vi "Run Action_Do.vi"(8 "error in (no error)":errorcluster, 10 "Project Builder in":refnum<class "Project Builder.lvclass">, 11 "Build Named Build Specification":refnum<class "Build Named Build Specification.lvclass">) -> (0 "error out":errorcluster, 1 "Success?":bool, 3 "Report":refnum<class "Report Data.lvclass">)   [LabVIEW 2019, in "ProjectBuilder.lvlib" / "Build Named Build Specification.lvclass"]
doc: "Run the action associated with the 'Project Action'-class.\n\nThis implementation builds a named build specification on the given target in the project."
uses:
  Build Named Build Specification.lvclass
  <vilib>/AppBuilder/AB_API_Simple/NI_App_Builder_API.lvlib
  Project Action/Project Action.lvclass
  Build Named Build Specification Data/Build Named Build Specification Data.lvclass
  <vilib>/AppBuilder/AB_API_Simple/Build (path).vi
  Data/Report Data/Report Data.lvclass
  Project Builder/Project Builder.lvclass
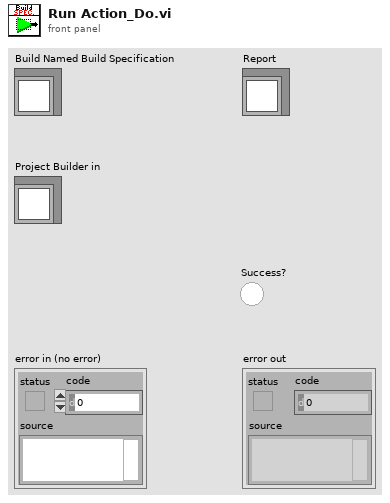
[diagram p1: front panel]
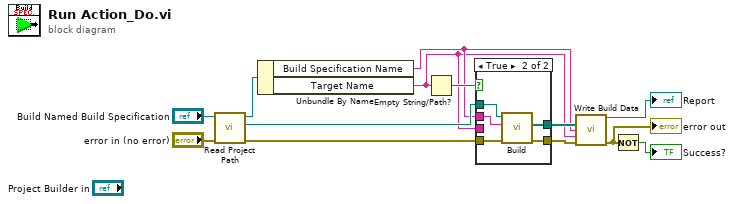
[diagram p0: block diagram]
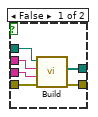
[diagram p2: hidden frame]
diagram:
  n1 = call "Read Project Path.vi"("error in (no error)"="error in (no error)", "Project Action in"="Build Named Build Specification") -> ("error out"=w9:errorcluster, "Project Path"=w10:path, "Project Action out"=w11:refnum<class "Build Named Build Specification.lvclass">)  [unwired: 7 in]
  n2 = Unbundle By Name(w11) -> ("Build Specification Name"=w2:string, "Target Name"=w1:string)
  n3 = Empty String/Path?(string/path=w1) -> (empty?=w4:bool)
  n4 = case shown="True" w4 {
    tunnel: w10 -> [w19 w24]
    tunnel: w2 -> [w18 w23]
    tunnel: w1 -> [w17 _]
    tunnel: w9 -> [w16 w22]
    tunnel: [w15 w21] -> w7
    tunnel: [w14 w20] -> w5
    frame False {
      n5 = call-poly <vilib>:"Build.vi"("error in (no error)"=w16, "Name of target (My Computer)"=w17, "Name of build specification (if empty: build all)"=w18, "Path to project"=w19) -> ("error out"=w15:errorcluster, "Generated files"=w14:path[])  [unwired: 6 in]
    }
    frame True {
      n6 = call-poly <vilib>:"Build.vi"("error in (no error)"=w22, "Name of build specification (if empty: build all)"=w23, "Path to project"=w24) -> ("error out"=w21:errorcluster, "Generated files"=w20:path[])  [unwired: 7 in]
    }
  }
  n7 = call "Write Build Data.vi"("Generated files"=w5, "Build Specification Name"=w2, "Target Name"=w1, "error in (no error)"=w7) -> ("Build Named Build Specification Data out"=→"Report":refnum<class "Build Named Build Specification Data.lvclass">, "error out"=w6:errorcluster)  [unwired: 10 in]
  "error out" <- w6
  n8 = Not(x=w6) -> (.not. x?=→"Success?":bool)
